vi "Initialize Protection Frames Outgoing.vi"(8 "error in (no error)":errorcluster, 10 "Frames":T1[](array[typedef]) {"Protection Configurations"."CRC Channels"."Data Type" items=["Signed", "Unsigned", "IEEE Float"]}, 11 "PCL (usec)":u32) -> (0 "error out":errorcluster, 2 "RT Frames":T8[](array[typedef]) {"Protection Configurations"."CRC Channels"."Data Type" items=["Signed", "Unsigned", "IEEE Float"]})   [LabVIEW 2019, in "Protection and Counter Support Engine.lvlib"]
uses:
  Protection and Counter Support Engine.lvlib
  Types/RT Frame Settings.ctl
  Shared/Types/Exported Frame Type.ctl
  Types/RT Protection Configuration.ctl
  Shared/Types/Protection Type.ctl
  Shared/Types/XNET Signal Configuration.ctl
  Shared/Types/Exported Counter Settings.ctl
  Shared/Types/Exported Event Trigger Type.ctl
  Shared/Types/Exported Frame Settings.ctl
  Shared/Types/Exported Protection Settings.ctl
  <vilib>/xnet/xnet.llb/XNET Create Session (Conversion).vi
  Shared/Protection and Counter Support Shared.lvlib
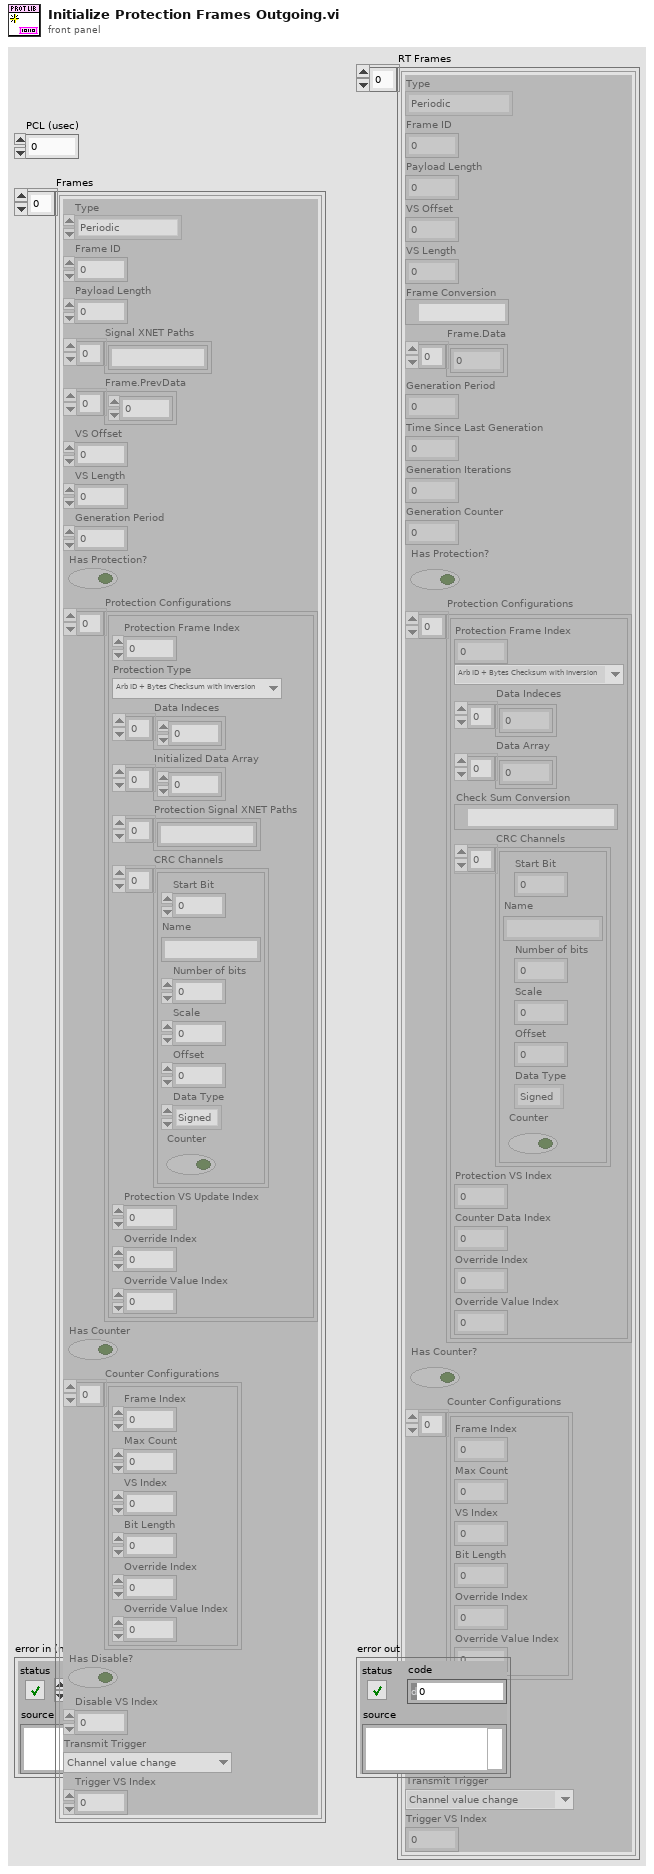
[diagram p1: front panel]
types:
  T1 = typedef "Protection and Counter Support Shared.lvlib/Exported Frame Settings.ctl" = cluster{"Type":T2, "Frame ID":u32, "Payload Length":u32, "Signal XNET Paths":string[], "Frame.PrevData":dbl[], "VS Offset":i32, "VS Length":i32, "Generation Period":u32, "Has Protection?":bool, "Protection Configurations":T3[], "Has Counter":bool, "Counter Configurations":T6[], "Has Disable?":bool, "Disable VS Index":i32, "Transmit Trigger":T7, "Trigger VS Index":i32}
  T2 = typedef "Protection and Counter Support Shared.lvlib/Exported Frame Type.ctl" = enum16{"Periodic", "Event", "Periodic/Event"}
  T3 = typedef "Protection and Counter Support Shared.lvlib/Exported Protection Settings.ctl" = cluster{"Protection Frame Index":i32, "Protection Type":T4, "Data Indeces":i32[], "Initialized Data Array":dbl[], "Protection Signal XNET Paths":string[], "CRC Channels":T5[], "Protection VS Update Index":i32, "Override Index":i32, "Override Value Index":i32}
  T4 = typedef "Protection and Counter Support Shared.lvlib/Protection Type.ctl" = enum16{"Arb ID + Bytes Checksum with Inversion", "Arb ID + Bytes CRC with Inversion", "Reversed Raw Signal Checksum with Inversion", "Concatenated Two's Compliment"}
  T5 = typedef "Protection and Counter Support Shared.lvlib/XNET Signal Configuration.ctl" = cluster{"Start Bit":i32, "Name":string, "Number of bits":i32, "Scale":dbl, "Offset":dbl, "Data Type":u32, "Counter":bool}
  T6 = typedef "Protection and Counter Support Shared.lvlib/Exported Counter Settings.ctl" = cluster{"Frame Index":i32, "Max Count":dbl, "VS Index":i32, "Bit Length":i64, "Override Index":i32, "Override Value Index":i32}
  T7 = typedef "Protection and Counter Support Shared.lvlib/Exported Event Trigger Type.ctl" = enum16{"Channel value change", "Trigger channel (not zero)", "Channel value change or trigger channel (not zero)", "Trigger channel (any value change)", "Channel value change or trigger channel (any value change)"}
  T8 = typedef "Protection and Counter Support Engine.lvlib/RT Frame Settings.ctl" = cluster{"Type":T2, "Frame ID":u32, "Payload Length":u32, "VS Offset":i32, "VS Length":i32, "Frame Conversion":refnum<k21>, "Frame.Data":dbl[], "Generation Period":u32, "Time Since Last Generation":u32, "Generation Iterations":u32, "Generation Counter":u32, "Has Protection?":bool, "Protection Configurations":T9[], "Has Counter?":bool, "Counter Configurations":T6[], "Has Disable?":bool, "Disable VS Index":i32, "Transmit Trigger":T7, "Trigger VS Index":i32}
  T9 = typedef "Protection and Counter Support Engine.lvlib/RT Protection Configuration.ctl" = cluster{"Protection Frame Index":i32, "Protection Type":T4, "Data Indeces":i32[], "Data Array":dbl[], "Check Sum Conversion":refnum<k21>, "CRC Channels":T5[], "Protection VS Index":i32, "Counter Data Index":i32, "Override Index":i32, "Override Value Index":i32}
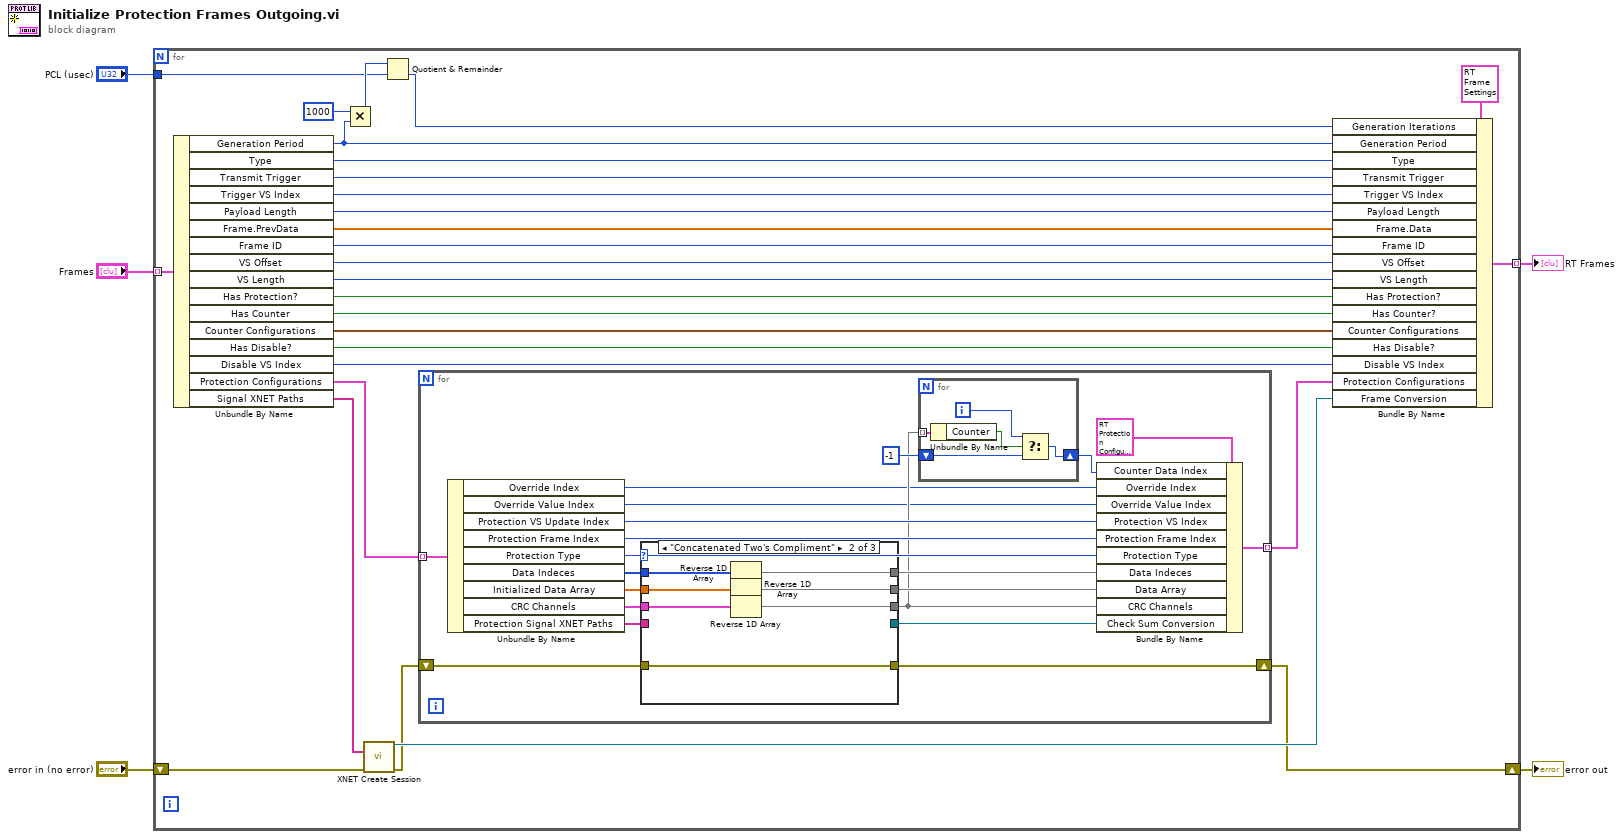
[diagram p0: block diagram]
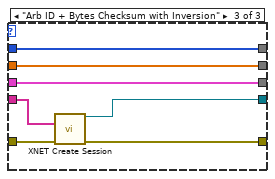
[diagram p3: hidden frame]
diagram:
  n1 = for {
    shift-right: [w18] -> w3
    shift-left: "error in (no error)" -> [w31]
    tunnel: "Frames" -> [w33] mode=indexing
    tunnel: [w17] -> w1 mode=indexing
    tunnel: "PCL (usec)" -> [w12]
    n2 = Unbundle By Name(w33) -> ("Generation Period"=w11:u32, "Type"=w6:T2, "Transmit Trigger"=w7:T7, "Trigger VS Index"=w8:i32, "Payload Length"=w9:u32, "Frame.PrevData"=w15:dbl[], "Frame ID"=w29:u32, "VS Offset"=w28:i32, "VS Length"=w27:i32, "Has Protection?"=w26:bool, "Has Counter"=w25:bool, "Counter Configurations"=w24:T6[], "Has Disable?"=w23:bool, "Disable VS Index"=w22:i32, "Protection Configurations"=w21:T3[], "Signal XNET Paths"=w32:string[])
    n3 = Multiply(x=u32 1000, y=w11) -> (x*y=w13:u32)
    n4 = call-poly <vilib>:"XNET Create Session.vi"("signal list"=w32, "error in (no error)"=w31) -> ("session out"=w30:refnum<k21>, "error out"=w19:errorcluster)  [unwired: 12 out]
    n5 = Quotient & Remainder(x=w13, y=w12) -> (floor(x/y)=w10:u32)  [unwired: 1 out]
    n6 = for {
      tunnel: w21 -> [w53] mode=indexing
      tunnel: [w48] -> w20 mode=indexing
      shift-right: [w46] -> w18
      shift-left: w19 -> [w47]
      n7 = Unbundle By Name(w53) -> ("Override Index"=w35:i32, "Override Value Index"=w34:i32, "Protection VS Update Index"=w37:i32, "Protection Frame Index"=w51:i32, "Protection Type"=w43:T4, "Data Indeces"=w38:i32[], "Initialized Data Array"=w40:dbl[], "CRC Channels"=w42:T5[], "Protection Signal XNET Paths"=w50:string[])
      n8 = case shown="\"Concatenated Two's Compliment\"" w43 {
        tunnel: w50 -> [_ _ w71]
        tunnel: [_ _ w70] -> w49
        tunnel: w47 -> [w57 w64 w69]
        tunnel: [w57 w64 w68] -> w46
        tunnel: [w56 w60 w67] -> w36
        tunnel: w42 -> [w56 w63 w67]
        tunnel: [w55 w59 w66] -> w41
        tunnel: w40 -> [w55 w62 w66]
        tunnel: [w54 w58 w65] -> w39
        tunnel: w38 -> [w54 w61 w65]
        frame Default {
        }
        frame "Concatenated Two's Compliment" {
          n9 = Reverse 1D Array(array=w61) -> (reversed array=w58:i32[])
          n10 = Reverse 1D Array(array=w62) -> (reversed array=w59:dbl[])
          n11 = Reverse 1D Array(array=w63) -> (reversed array=w60:T5[])
        }
        frame "Arb ID + Bytes Checksum with Inversion" {
          n12 = call-poly <vilib>:"XNET Create Session.vi"("signal list"=w71, "error in (no error)"=w69) -> ("session out"=w70:refnum<k21>, "error out"=w68:errorcluster)  [unwired: 12 out]
        }
      }
      n13 = for {
        tunnel: w36 -> [w76] mode=indexing
        shift-right: [w72] -> w44
        shift-left: -1 -> [w74]
        i -> [w73]
        n14 = Unbundle By Name(w76) -> ("Counter"=w75:bool)
        n15 = Select(t=w73, s=w75, f=w74) -> (s? t:f=w72:i32)
      }
      n16 = Bundle By Name(cluster=T9 {"Protection Frame Index"=0, "Protection Type"=enum."Arb ID + Bytes Checksum with Inversion", "Data Indeces"=[], "Data Array"=[], "Check Sum Conversion"="", "CRC Channels"=[], "Protection VS Index"=0, "Counter Data Index"=0, "Override Index"=0, "Override Value Index"=0} ("Cluster"), "Counter Data Index"=w44, "Override Index"=w35, "Override Value Index"=w34, "Protection VS Index"=w37, "Protection Frame Index"=w51, "Protection Type"=w43, "Data Indeces"=w39, "Data Array"=w41, "CRC Channels"=w36, "Check Sum Conversion"=w49) -> (w48:T9)
    }
    n17 = Bundle By Name(cluster=T8 {"Type"=enum."Periodic", "Frame ID"=0, "Payload Length"=0, "VS Offset"=0, "VS Length"=0, "Frame Conversion"="", "Frame.Data"=[], "Generation Period"=0, "Time Since Last Generation"=0, "Generation Iterations"=0, "Generation Counter"=0, "Has Protection?"=FALSE, "Protection Configurations"=[], "Has Counter?"=FALSE, "Counter Configurations"=[], "Has Disable?"=FALSE, "Disable VS Index"=0, "Transmit Trigger"=enum."Channel value change", "Trigger VS Index"=0} ("Frame Settings"), "Generation Iterations"=w10, "Generation Period"=w11, "Type"=w6, "Transmit Trigger"=w7, "Trigger VS Index"=w8, "Payload Length"=w9, "Frame.Data"=w15, "Frame ID"=w29, "VS Offset"=w28, "VS Length"=w27, "Has Protection?"=w26, "Has Counter?"=w25, "Counter Configurations"=w24, "Has Disable?"=w23, "Disable VS Index"=w22, "Protection Configurations"=w20, "Frame Conversion"=w30) -> (w17:T8)
  }
  "RT Frames" <- w1
  "error out" <- w3
